vi "Kinesis - PPC - Continuous Scan.vi"() -> ()   [LabVIEW 2012]
uses:
  U:/Kinesis LabVIEW Website Examples/Thorlabs.MotionControl.Controls.dll
  Thorlabs.MotionControl.Controls.dll
  U:/Kinesis LabVIEW Website Examples/ThorLabs.MotionControl.Benchtop.PrecisionPiezoCLI.dll
  ThorLabs.MotionControl.Benchtop.PrecisionPiezoCLI.dll
panel:
  in  "SerialNumber":string
  in  "Delay Factor":u32
  in  "Scaling Factor":i32
  in  "stop":bool
  in  "BenchtopPrecisionPiezoControl":refnum<k24>(container)
  # "Notes:"
  # "- Ensure that the appropriate .DLLs are copied into your Project Folder. Check that the correct bit type are used depending on your version of LabVIEW\ni.e. 32-bit or 64-bit.\n\n\n\n\n\n\n\n\n\n\n\n\n\n\n- Open the example VI through the LabVIEW Project Explorer to correctly load the User Interface from Thorlabs.MotionControl.Controls.dll."
  # "Thorlabs Hardware: PPC101 - Amplified Piezo Controller\n\nDevices:\n- LPS710E - https://www.thorlabs.com/newgrouppage9.cfm?objectgroup_id=11303\n- PFM450E - https://www.thorlabs.com/newgrouppage9.cfm?objectgroup_ID=9862&pn=PFM450E\n- PGM1SE - https://www.thorlabs.com/newgrouppage9.cfm?objectgroup_id=12199&pn=PGM1SE/M \n\nDescription: This VI will enable you to connect to a PPC* controlled device & linearly increment the piezo position at a user specified delay & step size. This VI will step the stage forward 5000 steps & then backward 5000 steps.\n\nInstructions: \n1) Connect your PPC* device to your PC & ensure it is powered on & the Output Enabled. \nFor full device setup,please refer to the device manual.\n2) Enter the device serial number below.\n3) Enter a Delay Factor below. This will initiate a delay in milliseconds.\n4) Enter a Scaling Factor below.\n3) Click 'Run' in the LabVIEW Toolbar."
  # "Example Image of .NET Controller - VI opened via Project Explorer/ not opened via Project Explorer"
  # "VI Not Opened via Project Explorer"
  # "VI Opened via Project Explorer"
  # "- To explore the range of methods available, please visit the .NET API, included with your Kinesis software.\n\n- For tips on building your own VIs with Thorlabs Motion Control Hardware, please see our LabVIEW Guide here.\nhttps://www.thorlabs.com/newgrouppage9.cfm?objectgroup_id=10285"
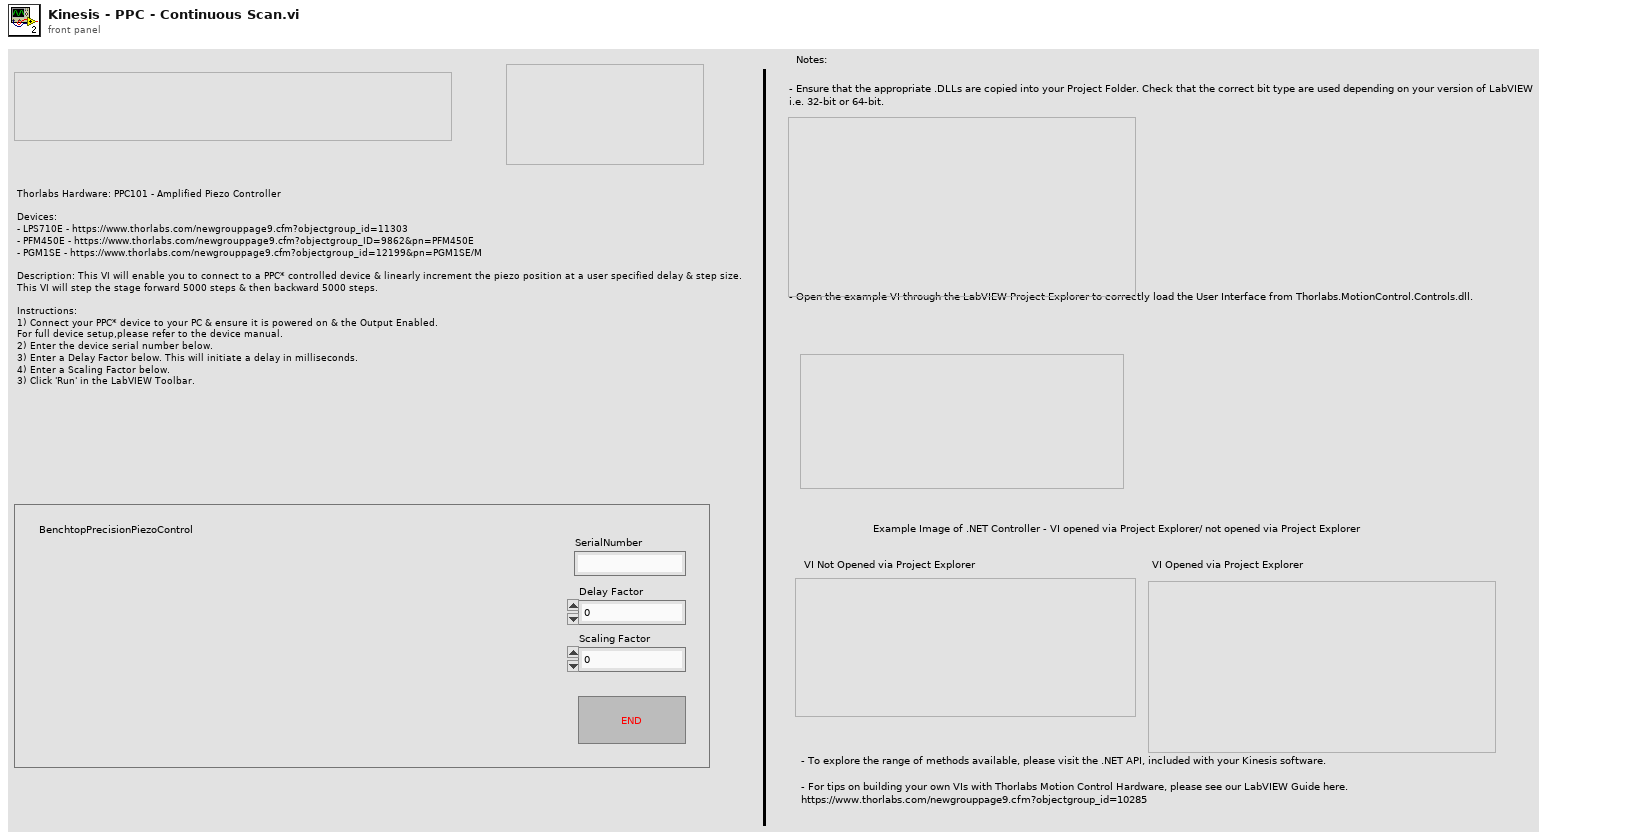
[diagram p1: front panel]
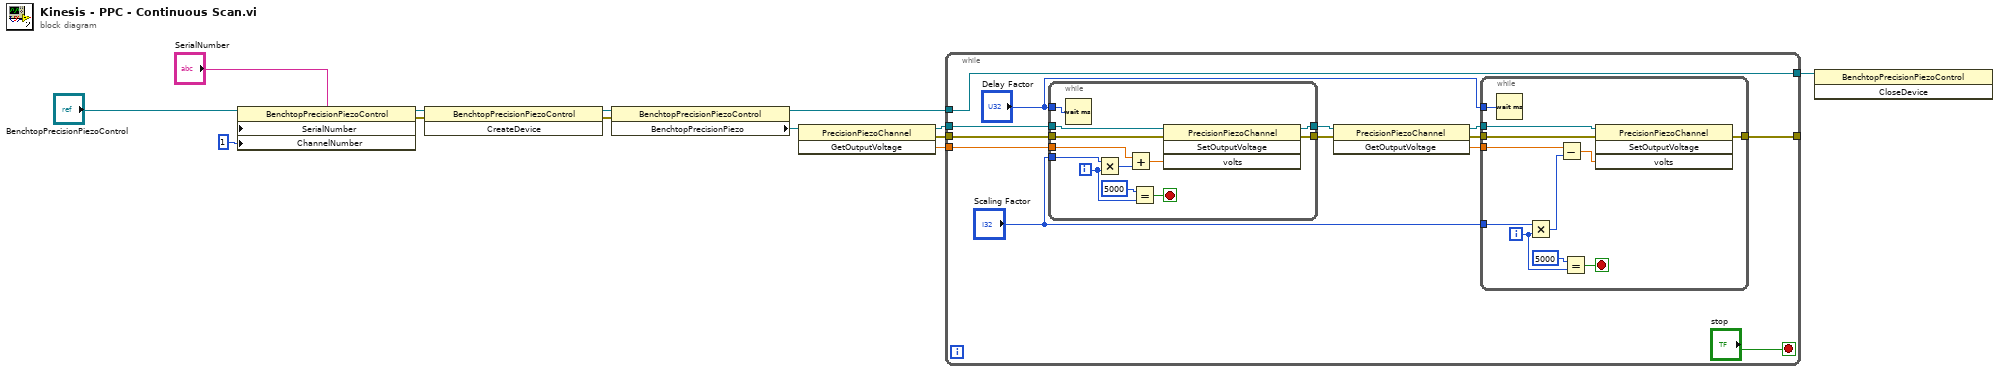
[diagram p0: block diagram]
diagram:
  n1 = property class="BenchtopPrecisionPiezoControl"(reference="BenchtopPrecisionPiezoControl", "SerialNumber"="SerialNumber", "ChannelNumber"=1) -> (reference out=w10:refnum<k24>, error out=w9:errorcluster)  [unwired: 1 in]
  n2 = invoke class="BenchtopPrecisionPiezoControl" method="CreateDevice"(reference=w10, error in=w9) -> (reference out=w12:refnum<k24>, error out=w11:errorcluster)  [unwired: 1 in, 1 out]
  n3 = property class="BenchtopPrecisionPiezoControl"(reference=w12, error in=w11) -> (reference out=w2:refnum<k24>, "BenchtopPrecisionPiezo"=w4:refnum<k24>)  [unwired: 1 out]
  n4 = invoke class="PrecisionPiezoChannel" method="GetOutputVoltage"(reference=w4) -> (reference out=w6:refnum<k24>, error out=w5:errorcluster, "GetOutputVoltage"=w7:dbl)  [unwired: 2 in]
  n5 = while {
    tunnel: w7 -> [w26]
    tunnel: w6 -> [w25]
    tunnel: w5 -> [w24]
    tunnel: [w17] -> _
    tunnel: [w14] -> w3
    tunnel: w2 -> [w14]
    stop <- "stop" stop-if-true
    n6 = while {
      tunnel: w26 -> [w47]
      tunnel: w25 -> [w44]
      tunnel: w24 -> [w42]
      tunnel: [w41] -> w23
      tunnel: [w40] -> w22
      tunnel: "Scaling Factor" -> [w39]
      tunnel: "Delay Factor" -> [w38]
      i -> [w46]
      stop <- w49 stop-if-true
      n7 = Wait (ms)(milliseconds to wait=w38) -> ()  [unwired: 1 out]
      n8 = Multiply(x=w39, y=w46) -> (x*y=w45:i32)
      n9 = Add(x=w47, y=w45) -> (x+y=w43:dbl)
      n10 = Equal?(x=5000, y=w46) -> (x = y?=w49:bool)
      n11 = invoke class="PrecisionPiezoChannel" method="SetOutputVoltage"(reference=w44, error in=w42, "volts"=w43) -> (reference out=w41:refnum<k24>, error out=w40:errorcluster)  [unwired: 1 in, 2 out]
    }
    n12 = invoke class="PrecisionPiezoChannel" method="GetOutputVoltage"(reference=w23, error in=w22) -> (reference out=w21:refnum<k24>, error out=w20:errorcluster, "GetOutputVoltage"=w19:dbl)  [unwired: 1 in]
    n13 = while {
      tunnel: w21 -> [w37]
      tunnel: w20 -> [w36]
      tunnel: w19 -> [w35]
      tunnel: [w29] -> w17
      tunnel: "Scaling Factor" -> [w28]
      tunnel: "Delay Factor" -> [w27]
      i -> [w32]
      stop <- w33 stop-if-true
      n14 = Wait (ms)(milliseconds to wait=w27) -> ()  [unwired: 1 out]
      n15 = Multiply(x=w28, y=w32) -> (x*y=w31:i32)
      n16 = Subtract(x=w35, y=w31) -> (x-y=w30:dbl)
      n17 = Equal?(x=5000, y=w32) -> (x = y?=w33:bool)
      n18 = invoke class="PrecisionPiezoChannel" method="SetOutputVoltage"(reference=w37, error in=w36, "volts"=w30) -> (error out=w29:errorcluster)  [unwired: 1 in, 3 out]
    }
  }
  n19 = invoke class="BenchtopPrecisionPiezoControl" method="CloseDevice"(reference=w3) -> ()  [unwired: 2 in, 3 out]
